vi "Init App Watcher.vi"(8 "error in (no error)":errorcluster, 11 "App in":refnum<class "App.lvclass">) -> (0 "error out":errorcluster, 3 "App out":refnum<class "App.lvclass">)   [LabVIEW 2020, in "PicoG-App.lvlib" / "App.lvclass"]
uses:
  App.lvclass
  App.lvclass/App.ctl
  App Watcher/App Watcher.lvclass
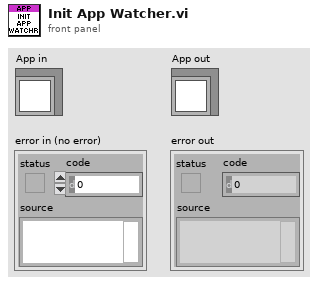
[diagram p1: front panel]
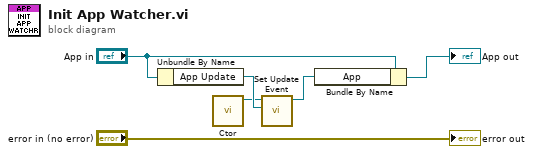
[diagram p0: block diagram]
diagram:
  n1 = Unbundle By Name("App in") -> ("App Update"=w3:refnum<user-event>)
  n2 = call "Ctor.vi"() -> ("App Watcher out"=w2:refnum<class "App Watcher.lvclass">)  [unwired: 10 in, 1 out]
  n3 = call "Set Update Event.vi"("App Update Event"=w3, "App Watcher in"=w2) -> ("App Watcher out"=w1:refnum<class "App Watcher.lvclass">)  [unwired: 8 in, 1 out]
  n4 = Bundle By Name(cluster="App in", "App"=w1) -> (→"App out":refnum<class "App.lvclass">)
  "error out" <- "error in (no error)"
